vi "FPGA tester without pulse width measurement.vi"(4 "error in":errorcluster, 5 "Delay":u32, 6 "Repetitions":dbl=1.0, 7 "Photon number":u16) -> (0 "error IO":errorcluster)   [LabVIEW 2013]
uses:
  <vilib>/DAQmx/write.llb/DAQmx Write (Digital Bool 1Line 1Point).vi
  <vilib>/DAQmx/read.llb/DAQmx Read (Digital Bool 1Line 1Point).vi
  <vilib>/DAQmx/miscellaneous.llb/DAQmx Fill In Error Info.vi
panel:
  in  "GPIB address":string="15"
  out "Set 1":bool[](array[boolean])
  out "Set 2":bool[](array[boolean])
  out "Set 3":bool[](array[boolean])
  out "Set 4":bool[](array[boolean])
  out "16-bit number":bool[](array[boolean])
  # "Or specify levels below:"
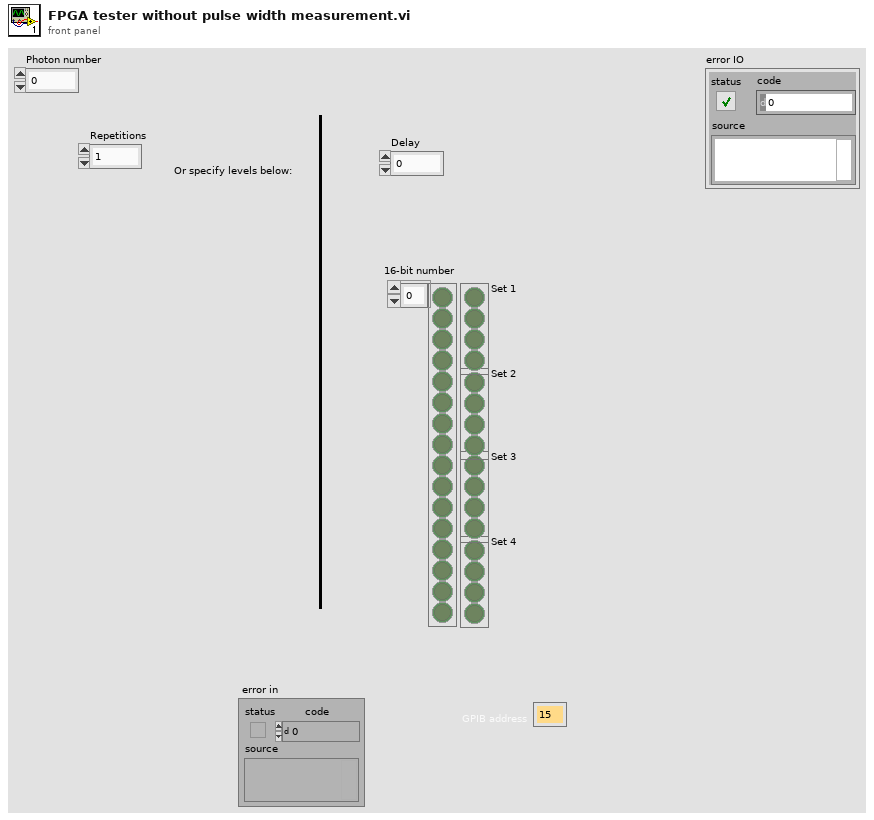
[diagram p1: front panel]
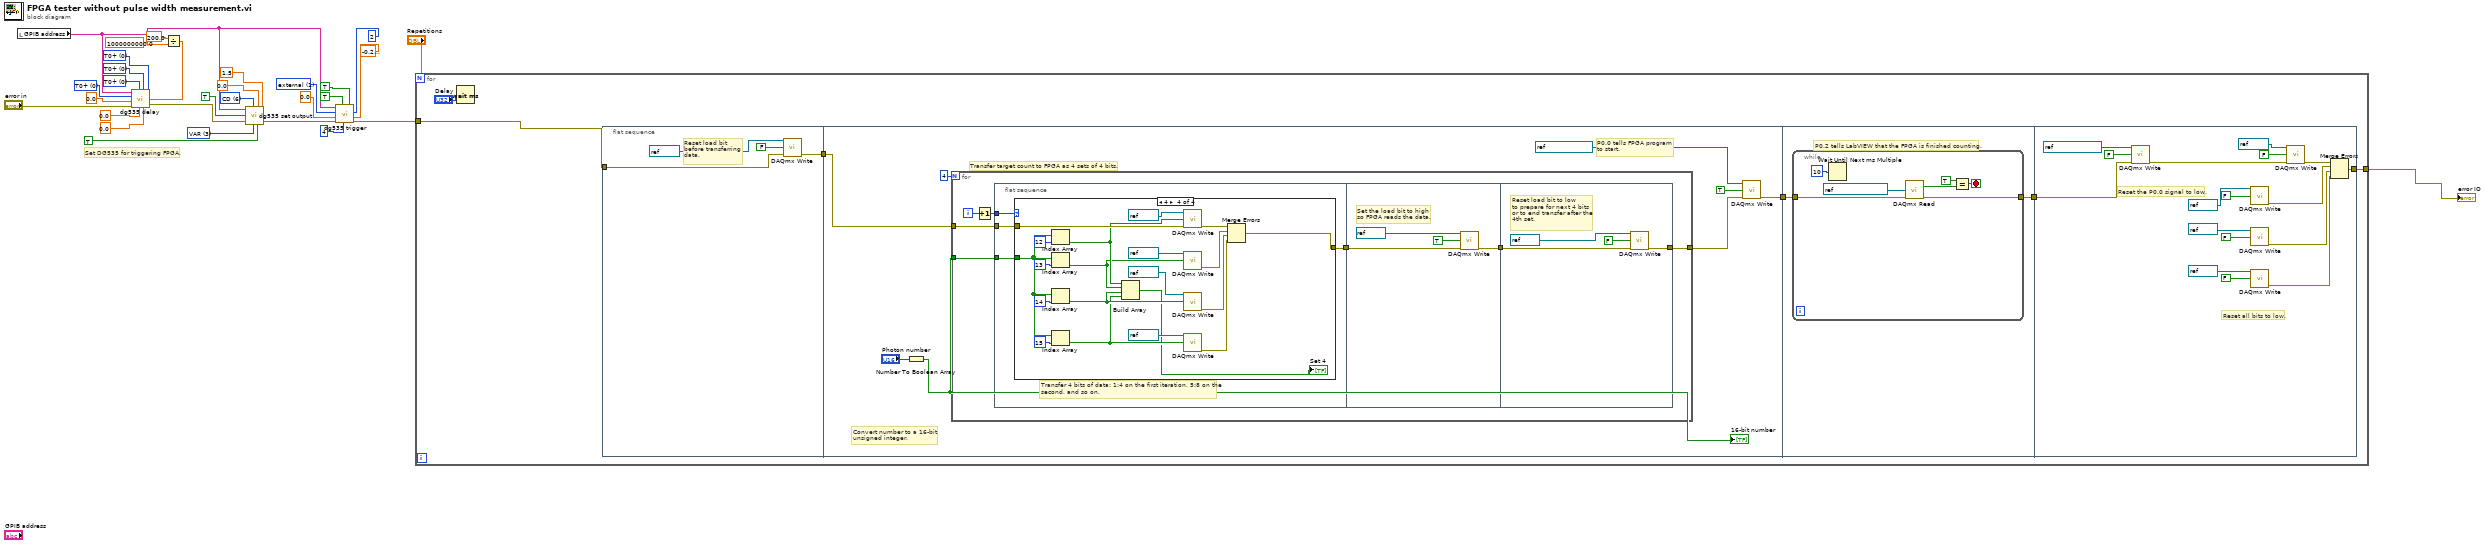
[diagram p0: block diagram]
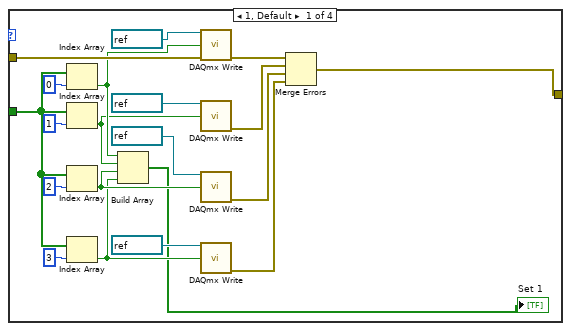
[diagram p2: hidden frame]
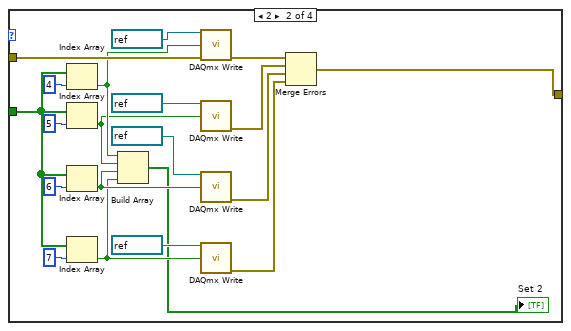
[diagram p3: hidden frame]
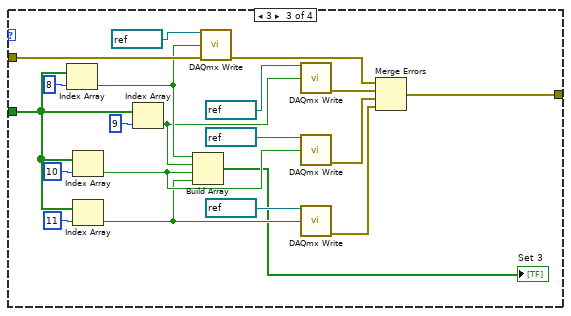
[diagram p4: hidden frame]
diagram:
  w19 = u32 1 items=["internal", "external", "single shot", "burst", "line"] ("trigger")
  w21 = 3 items=["TTL", "NIM", "ECL", "VAR"] ("mode")
  w23 = u16 6 items=["T0", "A", "B", "AB", "C", "D", "CD"] ("output")
  w26 = u32 0 items=["T0+", "A+", "B+", "C+"] ("D=")
  w27 = u32 0 items=["T0+", "A+", "B+", "D+"] ("C=")
  w28 = u32 0 items=["T0+", "A+", "C+", "D+"] ("B=")
  w29 = u32 0 items=["T0+", "B+", "C+", "D+"] ("A=")
  # "Set DG535 for triggering FPGA."
  n1 = local read "GPIB address"() -> (w11:string)
  n2 = Divide(x=200.0 ("D"), y=1000000000.0) -> (x/y=w5:dbl)
  n3 = call "dg535 delay.vi"("C"=0.0, "D"=w5, "D="=w26, "C="=w27, "B"=0.0 ("C"), "error in"="error in", "A"=0.0 ("D"), "B="=w28, "A="=w29, "GPIB address"=w11) -> ("error out"=w25:errorcluster)
  n4 = call "dg535 set output.vi"("GPIB address"=w11, "output"=w23, "set"=TRUE, "error in"=w25, "mode"=w21, "offset"=0.0, "amplitude"=1.5, "load"=TRUE) -> ("error out"=w12:errorcluster)  [unwired: 1 in]
  n5 = call "dg535 trigger.vi"("external trigger level"=sgl -0.2, "burst count"=2, "trigger slope"=TRUE, "burst period"=4, "input impedance"=TRUE, "error in"=w12, "internal/burst trigger rate"=0.0, "trigger"=w19, "GPIB address"=w11) -> ("error out"=w4:errorcluster)
  n6 = for {
    N: "Repetitions" -> [_]
    tunnel: w4 -> [w31]
    tunnel: [w32] -> w1
    n7 = Wait (ms)(milliseconds to wait="Delay") -> ()  [unwired: 1 out]
    n8 = flat-sequence {
      tunnel: w31 -> [w38]
      tunnel: [w37] -> w36
      tunnel: [w43] -> w35
      tunnel: w36 -> [w47]
      tunnel: w35 -> [w149]
      tunnel: [w148] -> w34
      tunnel: [w157] -> w32
      tunnel: w34 -> [w163]
      frame #0 {
        # "Reset load bit\nbefore transferring\ndata."
        n9 = call-poly <vilib>:"DAQmx Write.vi"("task/channels in"=refnum<k21> "BIT5", "data"=FALSE, "error in"=w38) -> ("error out"=w37:errorcluster)  [unwired: 10 in, 2 out]
      }
      frame #1 {
        # "P0.0 tells FPGA program \nto start."
        # "Convert number to a 16-bit\nunsigned integer."
        # "Transfer target count to FPGA as 4 sets of 4 bits."
        n10 = Number To Boolean Array(number="Photon number") -> (Boolean array=w42:bool[])
        "16-bit number" <- w42
        n11 = for {
          N: 4 -> [_]
          tunnel: w42 -> [w52]
          tunnel: w47 -> [w54]
          tunnel: [w49] -> w44
          i -> [w55]
          n12 = Increment(x=w55) -> (x+1=w53:i32)
          n13 = flat-sequence {
            tunnel: w54 -> [w59]
            tunnel: w53 -> [w58]
            tunnel: w52 -> [w57]
            tunnel: [w56] -> w51
            tunnel: w51 -> [w141]
            tunnel: [w140] -> w50
            tunnel: w50 -> [w145]
            tunnel: [w144] -> w49
            frame #0 {
              # "Transfer 4 bits of data: 1:4 on the first iteration, 5:8 on the\nsecond, and so on."
              n14 = case shown="4" w58 {
                tunnel: w57 -> [w67 w87 w107 w127]
                tunnel: w59 -> [w66 w86 w106 w126]
                tunnel: [w65 w85 w105 w125] -> w56
                frame 1, Default {
                  n15 = Index Array(array=w67, index=0) -> (element=w64:bool)
                  n16 = Index Array(array=w67, index=1) -> (element=w63:bool)
                  n17 = Index Array(array=w67, index=2) -> (element=w62:bool)
                  n18 = Index Array(array=w67, index=3) -> (element=w61:bool)
                  n19 = Build Array(w64, w63, w62, w61) -> (→"Set 1":bool[])
                  n20 = call-poly <vilib>:"DAQmx Write.vi"("task/channels in"=refnum<k21> "BIT1", "data"=w64, "error in"=w66) -> ("error out"=w75:errorcluster)  [unwired: 10 in, 2 out]
                  n21 = call-poly <vilib>:"DAQmx Write.vi"("task/channels in"=refnum<k21> "BIT2", "data"=w63) -> ("error out"=w74:errorcluster)  [unwired: 11 in, 2 out]
                  n22 = call-poly <vilib>:"DAQmx Write.vi"("task/channels in"=refnum<k21> "BIT3", "data"=w62) -> ("error out"=w73:errorcluster)  [unwired: 11 in, 2 out]
                  n23 = call-poly <vilib>:"DAQmx Write.vi"("task/channels in"=refnum<k21> "BIT4", "data"=w61) -> ("error out"=w72:errorcluster)  [unwired: 11 in, 2 out]
                  n24 = Merge Errors(w75, w74, w73, w72) -> (w65:errorcluster)
                }
                frame 2 {
                  n25 = Index Array(array=w87, index=4) -> (element=w84:bool)
                  n26 = Index Array(array=w87, index=5) -> (element=w83:bool)
                  n27 = Index Array(array=w87, index=6) -> (element=w82:bool)
                  n28 = Index Array(array=w87, index=7) -> (element=w81:bool)
                  n29 = Build Array(w84, w83, w82, w81) -> (→"Set 2":bool[])
                  n30 = call-poly <vilib>:"DAQmx Write.vi"("task/channels in"=refnum<k21> "BIT1", "data"=w84, "error in"=w86) -> ("error out"=w95:errorcluster)  [unwired: 10 in, 2 out]
                  n31 = call-poly <vilib>:"DAQmx Write.vi"("task/channels in"=refnum<k21> "BIT2", "data"=w83) -> ("error out"=w94:errorcluster)  [unwired: 11 in, 2 out]
                  n32 = call-poly <vilib>:"DAQmx Write.vi"("task/channels in"=refnum<k21> "BIT3", "data"=w82) -> ("error out"=w93:errorcluster)  [unwired: 11 in, 2 out]
                  n33 = call-poly <vilib>:"DAQmx Write.vi"("task/channels in"=refnum<k21> "BIT4", "data"=w81) -> ("error out"=w92:errorcluster)  [unwired: 11 in, 2 out]
                  n34 = Merge Errors(w95, w94, w93, w92) -> (w85:errorcluster)
                }
                frame 3 {
                  n35 = Index Array(array=w107, index=8) -> (element=w104:bool)
                  n36 = Index Array(array=w107, index=10) -> (element=w102:bool)
                  n37 = Index Array(array=w107, index=11) -> (element=w101:bool)
                  n38 = Index Array(array=w107, index=9) -> (element=w103:bool)
                  n39 = Build Array(w104, w103, w102, w101) -> (→"Set 3":bool[])
                  n40 = call-poly <vilib>:"DAQmx Write.vi"("task/channels in"=refnum<k21> "BIT1", "data"=w104, "error in"=w106) -> ("error out"=w115:errorcluster)  [unwired: 10 in, 2 out]
                  n41 = call-poly <vilib>:"DAQmx Write.vi"("task/channels in"=refnum<k21> "BIT2", "data"=w103) -> ("error out"=w114:errorcluster)  [unwired: 11 in, 2 out]
                  n42 = call-poly <vilib>:"DAQmx Write.vi"("task/channels in"=refnum<k21> "BIT3", "data"=w102) -> ("error out"=w113:errorcluster)  [unwired: 11 in, 2 out]
                  n43 = call-poly <vilib>:"DAQmx Write.vi"("task/channels in"=refnum<k21> "BIT4", "data"=w101) -> ("error out"=w112:errorcluster)  [unwired: 11 in, 2 out]
                  n44 = Merge Errors(w115, w114, w113, w112) -> (w105:errorcluster)
                }
                frame 4 {
                  n45 = Index Array(array=w127, index=12) -> (element=w124:bool)
                  n46 = Index Array(array=w127, index=13) -> (element=w123:bool)
                  n47 = Index Array(array=w127, index=14) -> (element=w122:bool)
                  n48 = Index Array(array=w127, index=15) -> (element=w121:bool)
                  n49 = Build Array(w124, w123, w122, w121) -> (→"Set 4":bool[])
                  n50 = call-poly <vilib>:"DAQmx Write.vi"("task/channels in"=refnum<k21> "BIT1", "data"=w124, "error in"=w126) -> ("error out"=w135:errorcluster)  [unwired: 10 in, 2 out]
                  n51 = call-poly <vilib>:"DAQmx Write.vi"("task/channels in"=refnum<k21> "BIT2", "data"=w123) -> ("error out"=w134:errorcluster)  [unwired: 11 in, 2 out]
                  n52 = call-poly <vilib>:"DAQmx Write.vi"("task/channels in"=refnum<k21> "BIT3", "data"=w122) -> ("error out"=w133:errorcluster)  [unwired: 11 in, 2 out]
                  n53 = call-poly <vilib>:"DAQmx Write.vi"("task/channels in"=refnum<k21> "BIT4", "data"=w121) -> ("error out"=w132:errorcluster)  [unwired: 11 in, 2 out]
                  n54 = Merge Errors(w135, w134, w133, w132) -> (w125:errorcluster)
                }
              }
            }
            frame #1 {
              # "Set the load bit to high\nso FPGA reads the data."
              n55 = call-poly <vilib>:"DAQmx Write.vi"("task/channels in"=refnum<k21> "BIT5", "data"=TRUE, "error in"=w141) -> ("error out"=w140:errorcluster)  [unwired: 10 in, 2 out]
            }
            frame #2 {
              # "Reset load bit to low\nto prepare for next 4 bits\nor to end transfer after the\n4th set."
              n56 = call-poly <vilib>:"DAQmx Write.vi"("task/channels in"=refnum<k21> "BIT5", "data"=FALSE, "error in"=w145) -> ("error out"=w144:errorcluster)  [unwired: 10 in, 2 out]
            }
          }
        }
        n57 = call-poly <vilib>:"DAQmx Write.vi"("task/channels in"=refnum<k21> "LaserChannel", "data"=TRUE, "error in"=w44) -> ("error out"=w43:errorcluster)  [unwired: 10 in, 2 out]
      }
      frame #2 {
        # "P0.2 tells LabVIEW that the FPGA is finished counting."
        n58 = while {
          tunnel: w149 -> [w156]
          tunnel: [w155] -> w148
          stop <- w152 stop-if-true
          n59 = Wait Until Next ms Multiple(millisecond multiple=u32 10) -> ()  [unwired: 1 out]
          n60 = call-poly <vilib>:"DAQmx Read.vi"("task/channels in"=refnum<k21> "P02countSignal", "error in"=w156) -> ("data"=w153:bool, "error out"=w155:errorcluster)  [unwired: 11 in, 1 out]
          n61 = Equal?(x=TRUE, y=w153) -> (x = y?=w152:bool)
        }
      }
      frame #3 {
        # "Reset all bits to low."
        # "Reset the P0.0 signal to low."
        n62 = call-poly <vilib>:"DAQmx Write.vi"("task/channels in"=refnum<k21> "LaserChannel", "data"=FALSE, "error in"=w163) -> ("error out"=w162:errorcluster)  [unwired: 10 in, 2 out]
        n63 = call-poly <vilib>:"DAQmx Write.vi"("task/channels in"=refnum<k21> "BIT2", "data"=FALSE) -> ("error out"=w170:errorcluster)  [unwired: 11 in, 2 out]
        n64 = call-poly <vilib>:"DAQmx Write.vi"("task/channels in"=refnum<k21> "BIT3", "data"=FALSE) -> ("error out"=w169:errorcluster)  [unwired: 11 in, 2 out]
        n65 = call-poly <vilib>:"DAQmx Write.vi"("task/channels in"=refnum<k21> "BIT4", "data"=FALSE) -> ("error out"=w168:errorcluster)  [unwired: 11 in, 2 out]
        n66 = call-poly <vilib>:"DAQmx Write.vi"("task/channels in"=refnum<k21> "BIT1", "data"=FALSE, "error in"=w162) -> ("error out"=w171:errorcluster)  [unwired: 10 in, 2 out]
        n67 = Merge Errors(w171, w170, w169, w168) -> (w157:errorcluster)
      }
    }
  }
  "error IO" <- w1
